vi "vpp.vi"(1 "Y":dbl[](array[numeric])=[-15.0, -14.0, -15.0, -16.0, -14.0, -15.0, -13.0, -14.0, -13.0, -15.0, -16.0, -13.0, -12.0, -14.0, -14.0, -14.0, -13.0, -14.0, -12.0, -14.0, -15.0, -15.0, -14.0, -15.0, -13.0, -18.0, -12.0, -14.0, -13.0, -14.0, -15.0, -14.0, -14.0, -15.0, -14.0, -16.0, -14.0, -13.0, -12.0, -16.0, -13.0, -14.0, -12.0, -14.0, -13.0, -14.0, -12.0, -15.0, -12.0, -16.0, -11.0, -14.0, -13.0, -13.0, -14.0, -11.0, -12.0, -11.0, -13.0, -16.0, -15.0, -11.0] format="%.2f", 2 "X":dbl[](array[numeric])=[-25.0, -26.0, -24.0, -24.0, -24.0, -26.0, -26.0, -22.0, -24.0, -23.0, -21.0, -25.0, -24.0, -21.0, -25.0, -21.0, -24.0, -26.0, -23.0, -21.0, -25.0, -24.0, -23.0, -23.0, -27.0, -22.0, -23.0, -21.0, -23.0, -21.0, -20.0, -20.0, -20.0, -22.0, -16.0, -21.0, -16.0, -21.0, -20.0, -22.0, -22.0, -16.0, -22.0, -18.0, -21.0, -20.0, -19.0, -20.0, -19.0, -21.0, -21.0, -20.0, -21.0, -21.0, -20.0, -21.0, -21.0, -20.0, -21.0, -19.0, -20.0, -21.0] format="%.2f") -> (0 "Vpp":dbl=7.280109889280518 format="%.2f")   [LabVIEW 2017]
doc: "This VI Calculates the maximum peak-to-peak value of a signal having x and y components. It does not work for signals such as pure sine waves. All of the plotting is really for trouble shooting purposes and should be removed for performance."
panel:
  out "Iterations":i32
  out "error out":errorcluster
  in  "error in (no error)":errorcluster
  out "XY Graph":cluster{dbl[], dbl[]}[](graph)=[{[-3.0, -4.0, -2.0, -2.0, -2.0, -4.0, -4.0, 0.0, -2.0, -1.0, 1.0, -3.0, -2.0, 1.0, -3.0, 1.0, -2.0, -4.0, -1.0, 1.0, -3.0, -2.0, -1.0, -1.0, -5.0, 0.0, -1.0, 1.0, -1.0, 1.0, 2.0, 2.0, 2.0, 0.0, 6.0, 1.0, 6.0, 1.0, 2.0, 0.0, 0.0, 6.0, 0.0, 4.0, 1.0, 2.0, 3.0, 2.0, 3.0, 1.0, 1.0, 2.0, 1.0, 1.0, 2.0, 1.0, 1.0, 2.0, 1.0, 3.0, 2.0, 1.0], [3.0, 4.0, 3.0, 2.0, 4.0, 3.0, 5.0, 4.0, 5.0, 3.0, 2.0, 5.0, 6.0, 4.0, 4.0, 4.0, 5.0, 4.0, 6.0, 4.0, 3.0, 3.0, 4.0, 3.0, 5.0, 0.0, 6.0, 4.0, 5.0, 4.0, 3.0, 4.0, 4.0, 3.0, 4.0, 2.0, 4.0, 5.0, 6.0, 2.0, 5.0, 4.0, 6.0, 4.0, 5.0, 4.0, 6.0, 3.0, 6.0, 2.0, 7.0, 4.0, 5.0, 5.0, 4.0, 7.0, 6.0, 7.0, 5.0, 2.0, 3.0, 7.0]}, {[2.0], [7.0]}, {[-5.0], [5.0]}]
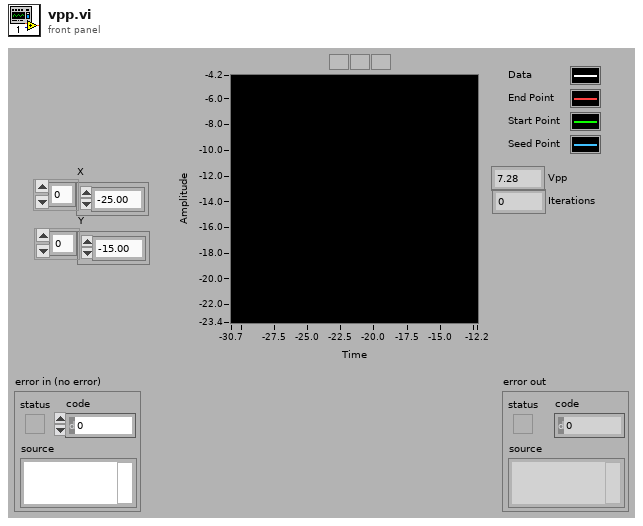
[diagram p1: front panel]
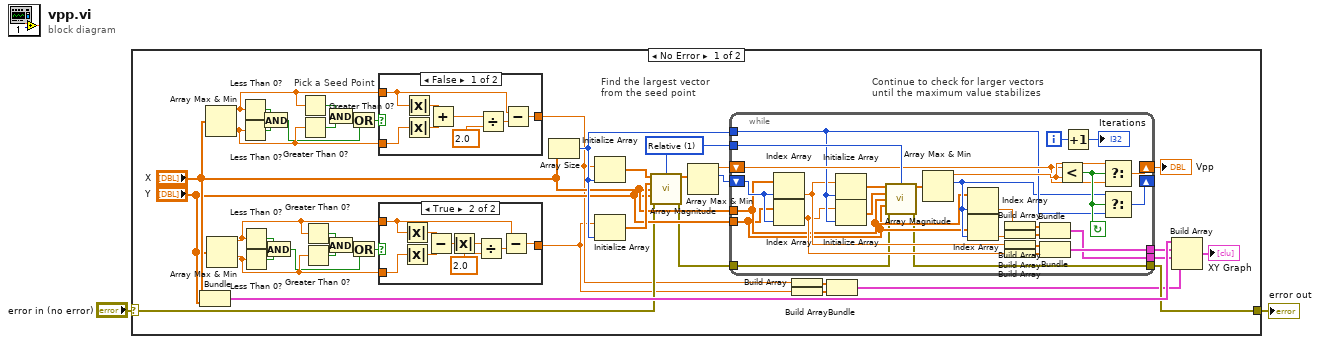
[diagram p0: block diagram]
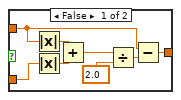
[diagram p2: hidden frame]
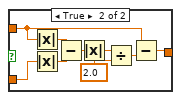
[diagram p3: hidden frame]
diagram:
  n1 = case shown="No Error" "error in (no error)" {
    selector: "error in (no error)" -> [w28 w105]
    tunnel: [w26 w105] -> w1
    frame No Error {
      w36 = u16 1 items=["Absolute", "Relative"] ("Mode")
      # "Continue to check for larger vectors\nuntil the maximum value stabilizes"
      # "Find the largest vector \nfrom the seed point"
      # "Pick a Seed Point"
      n2 = Bundle("X"="X", "Y"="Y") -> (w30:cluster{"X":dbl[], "Y":dbl[]})  [unwired: 1 in]
      n3 = Array Max & Min(array="X") -> (max value=w12:dbl, min value=w9:dbl)  [unwired: 2 out]
      n4 = Array Max & Min(array="Y") -> (max value=w5:dbl, min value=w4:dbl)  [unwired: 2 out]
      n5 = Less Than 0?(x=w12) -> (x < 0?=w22:bool)
      n6 = Less Than 0?(x=w9) -> (x < 0?=w21:bool)
      n7 = Less Than 0?(x=w5) -> (x < 0?=w18:bool)
      n8 = Less Than 0?(x=w4) -> (x < 0?=w19:bool)
      n9 = And(x=w22, y=w21) -> (x .and. y?=w8:bool)
      n10 = And(x=w18, y=w19) -> (x .and. y?=w3:bool)
      n11 = Greater Than 0?(x=w12) -> (x > 0?=w11:bool)
      n12 = Greater Than 0?(x=w9) -> (x > 0?=w10:bool)
      n13 = Greater Than 0?(x=w5) -> (x > 0?=w7:bool)
      n14 = Greater Than 0?(x=w4) -> (x > 0?=w6:bool)
      n15 = And(x=w11, y=w10) -> (x .and. y?=w14:bool)
      n16 = And(x=w7, y=w6) -> (x .and. y?=w13:bool)
      n17 = Or(x=w14, y=w8) -> (x .or. y?=w16:bool)
      n18 = Or(x=w13, y=w3) -> (x .or. y?=w15:bool)
      n19 = case shown="False" w16 {
        tunnel: w9 -> [w63 w70]
        tunnel: w12 -> [w61 w69]
        tunnel: [w62 w68] -> w20
        frame False {
          n20 = Absolute Value(x=w61) -> (abs(x)=w65:dbl)
          n21 = Absolute Value(x=w63) -> (abs(x)=w66:dbl)
          n22 = Add(x=w65, y=w66) -> (x+y=w60:dbl)
          n23 = Divide(x=w60, y=2.0) -> (x/y=w64:dbl)
          n24 = Subtract(x=w61, y=w64) -> (x-y=w62:dbl)
        }
        frame True {
          n25 = Absolute Value(x=w69) -> (abs(x)=w72:dbl)
          n26 = Absolute Value(x=w70) -> (abs(x)=w73:dbl)
          n27 = Subtract(x=w72, y=w73) -> (x-y=w75:dbl)
          n28 = Absolute Value(x=w75) -> (abs(x)=w76:dbl)
          n29 = Divide(x=w76, y=2.0) -> (x/y=w71:dbl)
          n30 = Subtract(x=w69, y=w71) -> (x-y=w68:dbl)
        }
      }
      n31 = case shown="True" w15 {
        tunnel: w4 -> [w46 w53]
        tunnel: w5 -> [w44 w52]
        tunnel: [w45 w51] -> w17
        frame False {
          n32 = Absolute Value(x=w44) -> (abs(x)=w48:dbl)
          n33 = Absolute Value(x=w46) -> (abs(x)=w49:dbl)
          n34 = Add(x=w48, y=w49) -> (x+y=w43:dbl)
          n35 = Divide(x=w43, y=2.0) -> (x/y=w47:dbl)
          n36 = Subtract(x=w44, y=w47) -> (x-y=w45:dbl)
        }
        frame True {
          n37 = Absolute Value(x=w52) -> (abs(x)=w55:dbl)
          n38 = Absolute Value(x=w53) -> (abs(x)=w56:dbl)
          n39 = Subtract(x=w55, y=w56) -> (x-y=w58:dbl)
          n40 = Absolute Value(x=w58) -> (abs(x)=w59:dbl)
          n41 = Divide(x=w59, y=2.0) -> (x/y=w54:dbl)
          n42 = Subtract(x=w52, y=w54) -> (x-y=w51:dbl)
        }
      }
      n43 = Array Size(array="X") -> (size(s)=w37:i32)
      n44 = Initialize Array(w20, w37) -> (w42:dbl[])
      n45 = Initialize Array(w17, w37) -> (w41:dbl[])
      n46 = call "Array Magnitude.vi"("x"=w42, "Mode"=w36, "y"=w41, "x 2"="X", "y 2"="Y", "error in (no error)"=w28) -> ("z"=w40:dbl[], "error out"=w27:errorcluster)  [unwired: 8 in]
      n47 = Array Max & Min(array=w40) -> (max value=w39:dbl, max index (indices)=w38:i32)  [unwired: 2 out]
      n48 = while {
        shift-right: [w99] -> w33
        shift-left: w39 -> [w95]
        tunnel: "X" -> [w88]
        tunnel: "Y" -> [w87]
        shift-right: [w97] -> _
        shift-left: w38 -> [w104]
        tunnel: w37 -> [w94]
        tunnel: w36 -> [w103]
        tunnel: [w82] -> w24
        tunnel: [w81] -> w23
        tunnel: w27 -> [w80]
        tunnel: [w79] -> w26
        i -> [w78]
        stop <- w98 continue-if-true
        n49 = Index Array(array=w88, index=w104) -> (element=w91:dbl)
        n50 = Index Array(array=w87, index=w104) -> (element=w90:dbl)
        n51 = Initialize Array(w91, w94) -> (w102:dbl[])
        n52 = Initialize Array(w90, w94) -> (w101:dbl[])
        n53 = call "Array Magnitude.vi"("x"=w102, "Mode"=w103, "y"=w101, "x 2"=w88, "y 2"=w87, "error in (no error)"=w80) -> ("z"=w100:dbl[], "error out"=w79:errorcluster)  [unwired: 8 in]
        n54 = Array Max & Min(array=w100) -> (max value=w96:dbl, max index (indices)=w89:i32)  [unwired: 2 out]
        n55 = Index Array(array=w88, index=w89) -> (element=w84:dbl)
        n56 = Index Array(array=w87, index=w89) -> (element=w83:dbl)
        n57 = Build Array(w84) -> (w86:dbl[])
        n58 = Build Array(w83) -> (w85:dbl[])
        n59 = Build Array(w91) -> (w92:dbl[])
        n60 = Build Array(w90) -> (w93:dbl[])
        n61 = Bundle(w86, w85) -> (w81:cluster{dbl[], dbl[]})  [unwired: 1 in]
        n62 = Bundle(w92, w93) -> (w82:cluster{dbl[], dbl[]})  [unwired: 1 in]
        n63 = Less?(x=w95, y=w96) -> (x < y?=w98:bool)
        n64 = Increment(x=w78) -> (x+1=→"Iterations":i32)
        n65 = Select(t=w96, s=w98, f=w95) -> (s? t:f=w99:dbl)
        n66 = Select(t=w89, s=w98, f=w94) -> (s? t:f=w97:i32)
      }
      "Vpp" <- w33
      n67 = Build Array(w20) -> (w34:dbl[])
      n68 = Build Array(w17) -> (w35:dbl[])
      n69 = Bundle(w34, w35) -> (w25:cluster{dbl[], dbl[]})  [unwired: 1 in]
      n70 = Build Array(w30, w24, w23, w25) -> (→"XY Graph":cluster{"X":dbl[], "Y":dbl[]}[])
    }
    frame Error {
    }
  }
  "error out" <- w1
